vi "Create Telemetry API.vi"(8 "error in (no error)":errorcluster, 11 "VolatusCore in":refnum<class "VolatusCore.lvclass">) -> (0 "error out":errorcluster, 3 "VolatusCore out":refnum<class "VolatusCore.lvclass">)   [LabVIEW 2020, in "Volatus.lvlib" / "VolatusCore.lvclass"]
uses:
  VolatusCore.lvclass
  VolatusCore.lvclass/VolatusCore.ctl
  TelemetryAPI/TelemetryAPI.lvclass
  lv-vecto/Vecto/Vecto/Vecto.lvclass
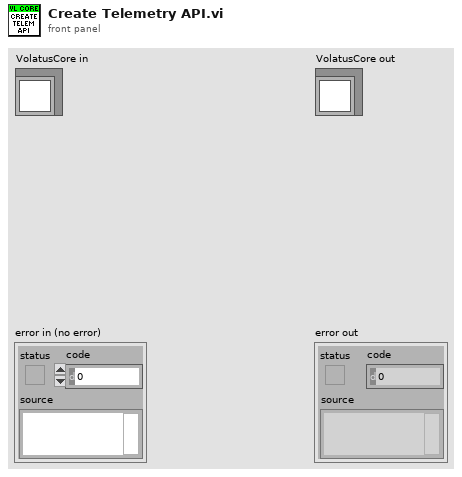
[diagram p1: front panel]
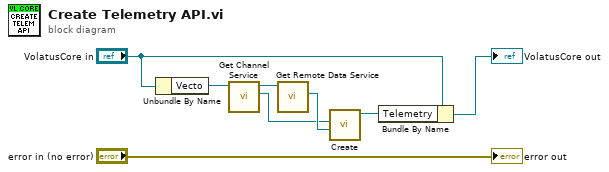
[diagram p0: block diagram]
diagram:
  n1 = Unbundle By Name("VolatusCore in") -> ("Vecto"=w1:refnum<class "Vecto.lvclass">)
  n2 = call "Get Channel Service.vi"("Vecto in"=w1) -> ("ChannelService"=w5:refnum<class "ChannelService.lvclass">, "Vecto out"=w7:refnum<class "Vecto.lvclass">)  [unwired: 8 in, 1 out]
  n3 = call "Get Remote Data Service.vi"("Vecto in"=w7) -> ("RemoteDataService"=w6:refnum<class "RemoteDataService.lvclass">)  [unwired: 8 in, 2 out]
  n4 = call "Create.vi"("RemoteDataService"=w6, "ChannelService"=w5) -> ("TelemetryAPI out"=w4:refnum<class "TelemetryAPI.lvclass">)  [unwired: 8 in, 1 out]
  n5 = Bundle By Name(cluster="VolatusCore in", "Telemetry"=w4) -> (→"VolatusCore out":refnum<class "VolatusCore.lvclass">)
  "error out" <- "error in (no error)"
